vi "Host_timing_study.vi"() -> ()   [LabVIEW 2020]
uses:
  <vilib>/Analysis/7linalg.llb/Eigenvalue and Vectors Output Option.ctl
  <vilib>/Analysis/NI_AALPro.lvlib
  <vilib>/Analysis/7linalg.llb/Real Eigenvalues and Vectors.vi
  <vilib>/Analysis/NI_AALBase.lvlib
  <vilib>/Analysis/baseanly.llb/Real Inverse Matrix.vi
  <vilib>/rvi/interface/nirviMethod/nirviMethod.xnode
  <vilib>/Analysis/Matrix/NI_Matrix.lvlib
  <vilib>/Analysis/Matrix/Numeric/Multiply/Multiply - RM,RM.vi
  <vilib>/rvi/errors/niLvFpgaMergeErrorWithErrorCode.vi
  <vilib>/rvi/interface/nirviOpenFPGA/nirviOpenFPGA.xnode
  <vilib>/rvi/interface/nirviCloseFPGA/nirviCloseFPGA.xnode
  <vilib>/FPGAPlugInAG/Dynamic/niLvFpga_Close_Dynamic.vi
  <vilib>/Analysis/baseanly.llb/Matrix Type of Inverse Matrix.ctl
  FPGA Bitfiles/Cholesky_SGL_19_nodes.lvbitx
  <vilib>/FPGAPlugInAG/Dynamic/niLvFpga_Run_Dynamic.vi
  <vilib>/Analysis/Matrix/Numeric/Add/Add - RM,RM.vi
  <vilib>/addons/Multicore Analysis and Sparse Matrix/Linear Algebra/_linalg/Eigenvalues and Vectors_Output Option.ctl
  <vilib>/addons/Multicore Analysis and Sparse Matrix/Linear Algebra/_linalg/Eigenvalues and Vectors_Matrix Type (Real).ctl
  <vilib>/addons/Multicore Analysis and Sparse Matrix/Linear Algebra/_linalg/Eigenvalues and Vectors (DBL).vi
  <vilib>/addons/Multicore Analysis and Sparse Matrix/Linear Algebra/_linalg/Inverse Matrix (DBL).vi
  <vilib>/addons/Multicore Analysis and Sparse Matrix/Linear Algebra/_linalg/Inverse Matrix_Matrix Type.ctl
  <vilib>/addons/Multicore Analysis and Sparse Matrix/Linear Algebra/_linalg/Transpose Matrix (DBL).vi
  <vilib>/Analysis/Matrix/Numeric/Conversions/Array To Matrix - RA2.vi
  <vilib>/addons/Multicore Analysis and Sparse Matrix/Linear Algebra/_linalg/Cholesky Decomposition (DBL).vi
  <vilib>/Analysis/7linalg.llb/Real Cholesky Factorization.vi
  <vilib>/addons/Multicore Analysis and Sparse Matrix/Linear Algebra/_linalg/Generalized Eigenvalues and Vectors (DBL).vi
  <vilib>/Analysis/7linalg.llb/Real Generalized Eigenvalues and Vectors.vi
  FPGA Bitfiles/cholesky_SGL_CCL_19_nodes_v3.lvbitx
  <vilib>/FPGAPlugInAG/Dynamic/niLvFpga_WriteFifo_Dynamic.vi
  <vilib>/FPGAPlugInAG/Dynamic/niLvFpga_ReadFifo_Dynamic.vi
panel:
  out "Data":sgl[](array[numeric])
  out "Real 2D Array":dbl[][](array[numeric])
  in  "Enum":T1(ring)
  out "Eigenvalues":cdb[](array[numeric])
  out "eigenvalue solver (ms)":dbl
  out "preprocessing (ms)":dbl
  out "total run time (ms)":dbl
  out "Frequencies":dbl[](array[numeric])
  out "K input":dbl[][](array[numeric])
  out "M input":dbl[][](array[numeric])
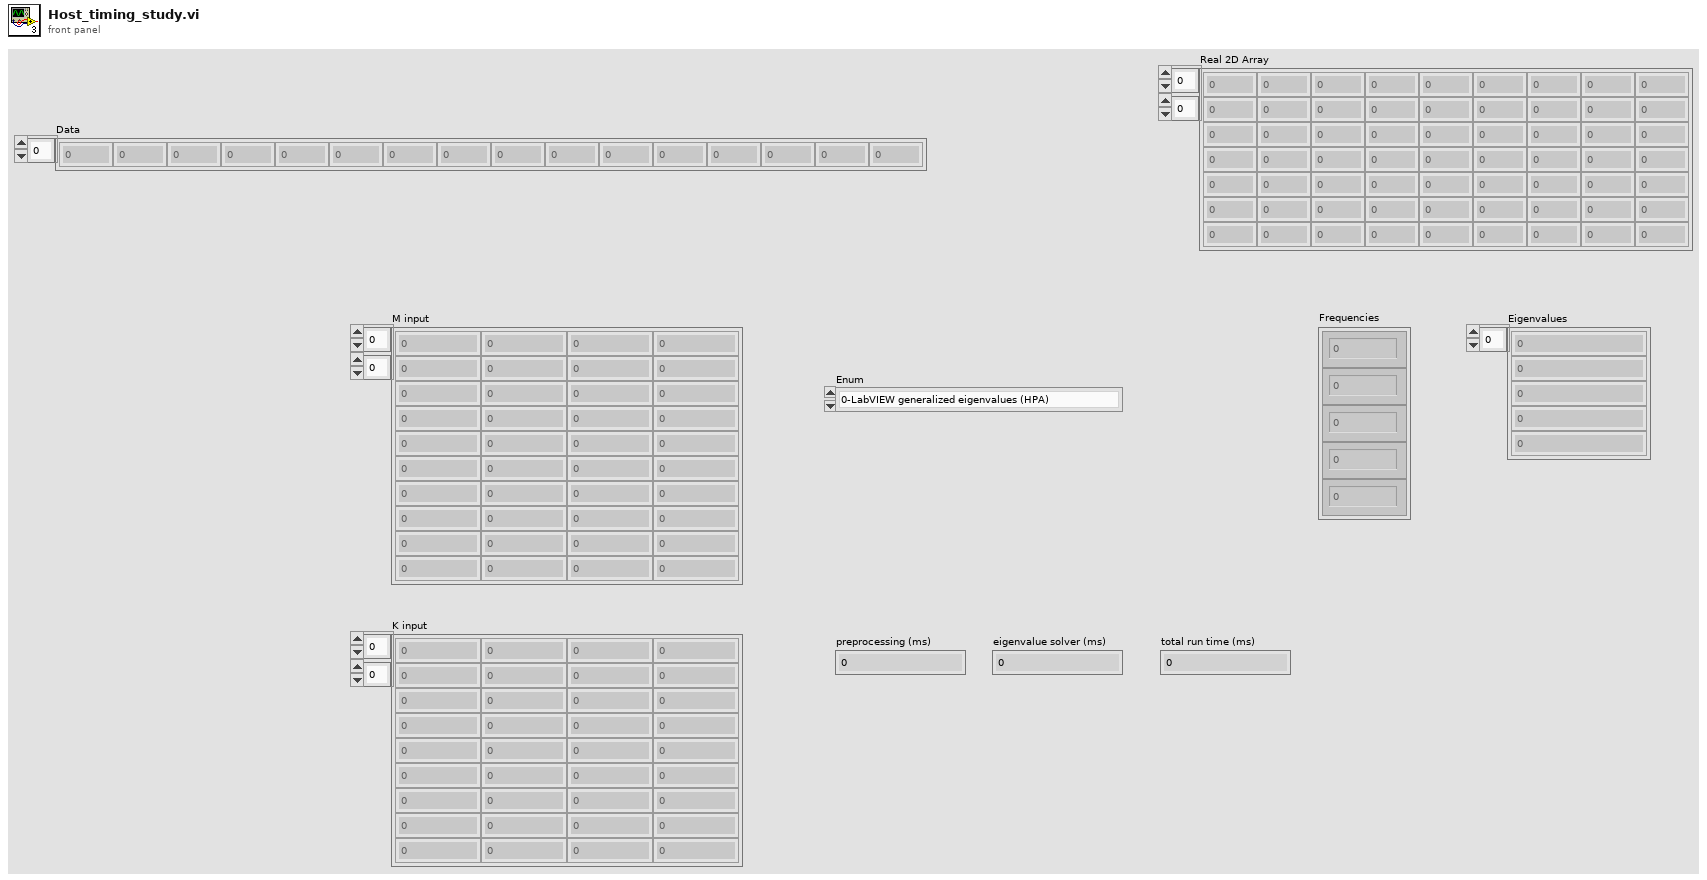
[diagram p1: front panel]
types:
  T1 = enum16{"0-LabVIEW generalized eigenvalues (HPA)", "1-LabVIEW generalized eigenvalues", "2-LabVIEW M^-1K eigenvalues (HPA)", "3-LabVIEW M^-1K eigenvalues", "4-LabVIEW Cholesky Factorization (HPA)", "5-LabVIEW Cholesky Factorization", "6-Cholesky Factorization CPU SGL", "7-Cholesky Factorization CPU FXP", "8-Cholesky Factorization FPGA SGL", "9-Cholesky Factorization FPGA SGL SCL"}
  T2 = typedef "NI_AALBase.lvlib/Matrix Type of Inverse Matrix.ctl" = enum32{"General", "Positive Definite", "Lower Triangular", "Upper Triangular"}
  T3 = typedef "NI_MASM_MtrxDecomposition.lvlib/Eigenvalues and Vectors_Output Option.ctl" = i32
  T4 = typedef "NI_Matrix.lvlib/RealMatrix.ctl" = dbl[][]
  T5 = typedef "NI_AALPro.lvlib/Eigenvalue and Vectors Output Option.ctl" = i32
  T6 = typedef "NI_MASM_BasicLinAlg.lvlib/Inverse Matrix_Matrix Type.ctl" = i32
  T7 = typedef "NI_MASM_MtrxDecomposition.lvlib/Eigenvalues and Vectors_Matrix Type (Real).ctl" = i32
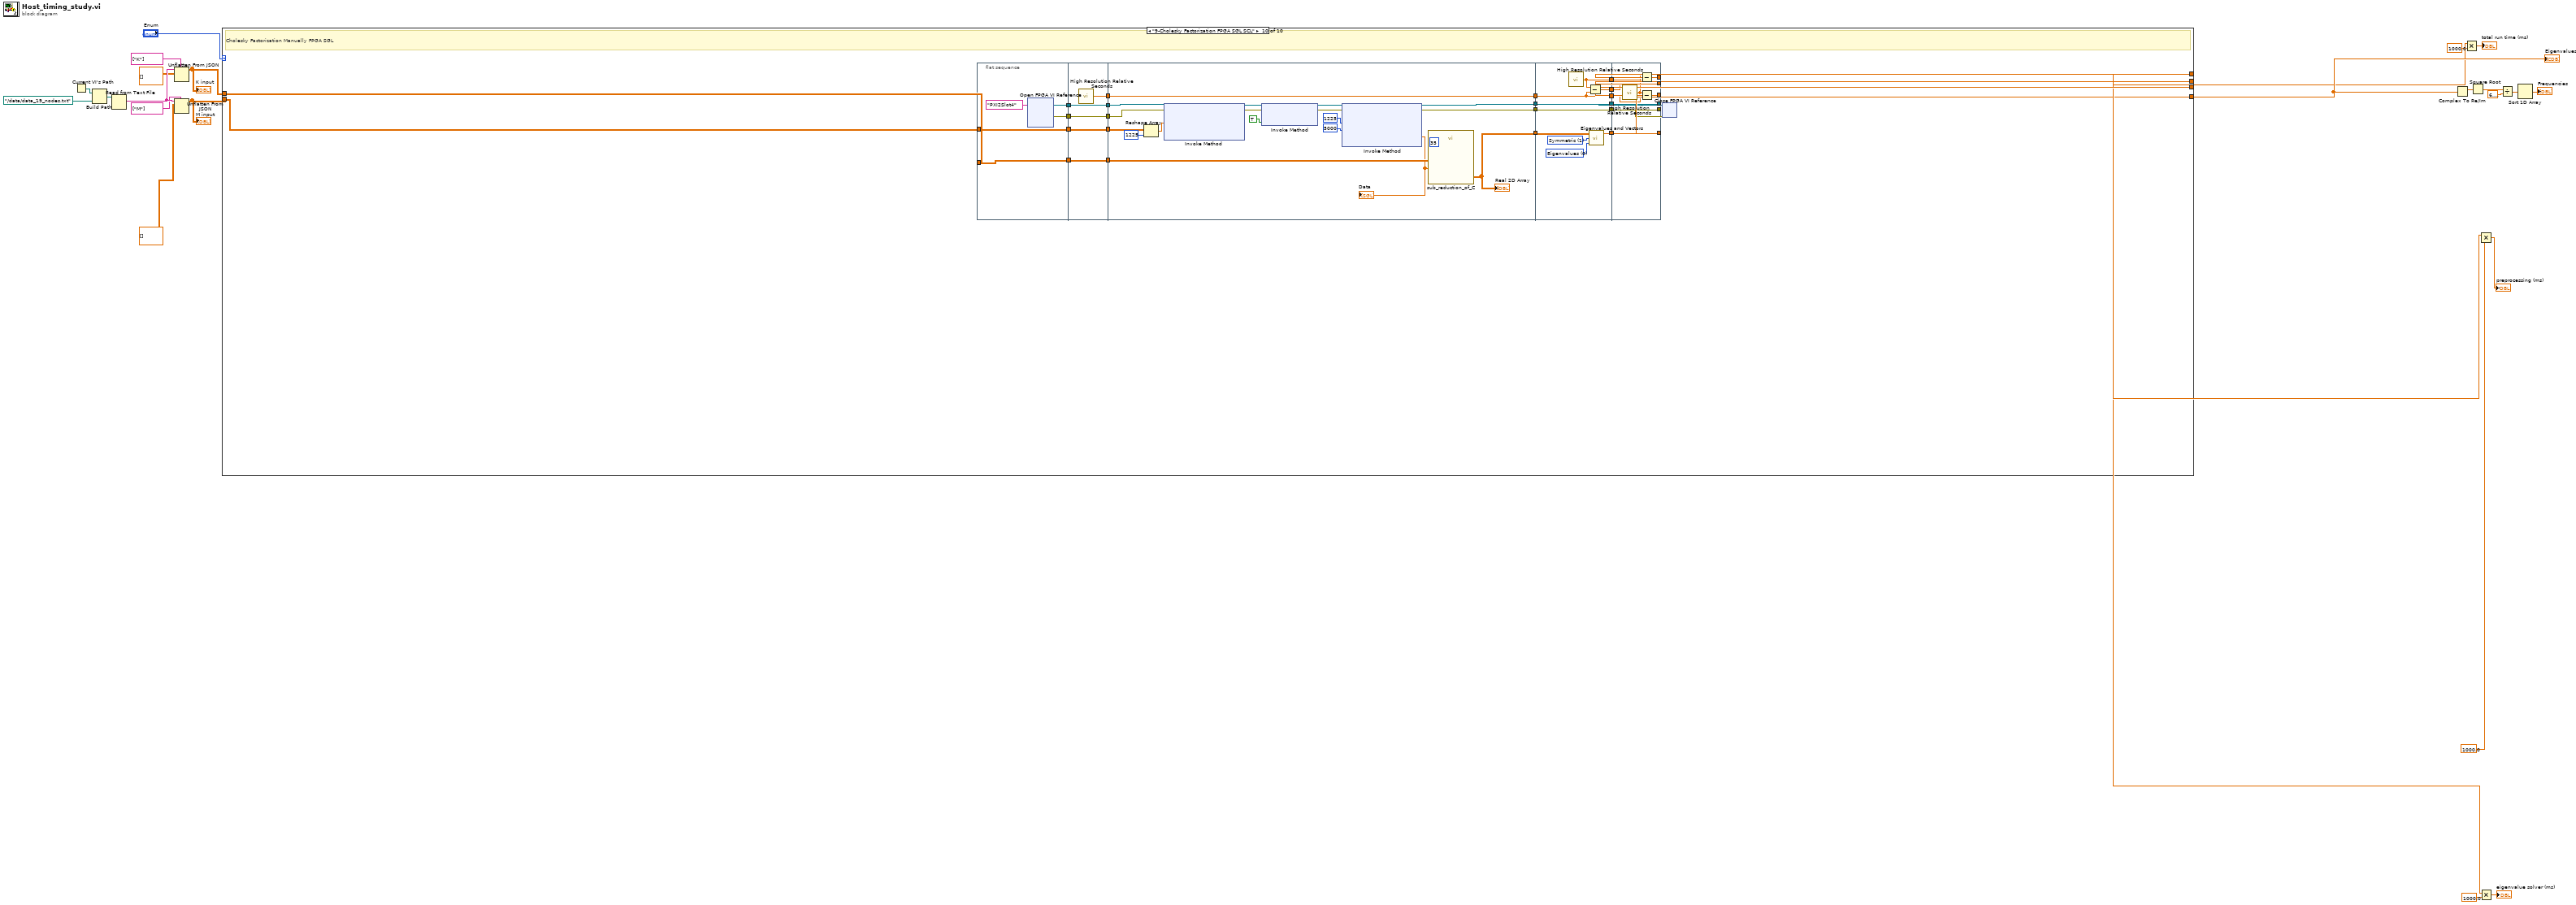
[diagram p0: block diagram]
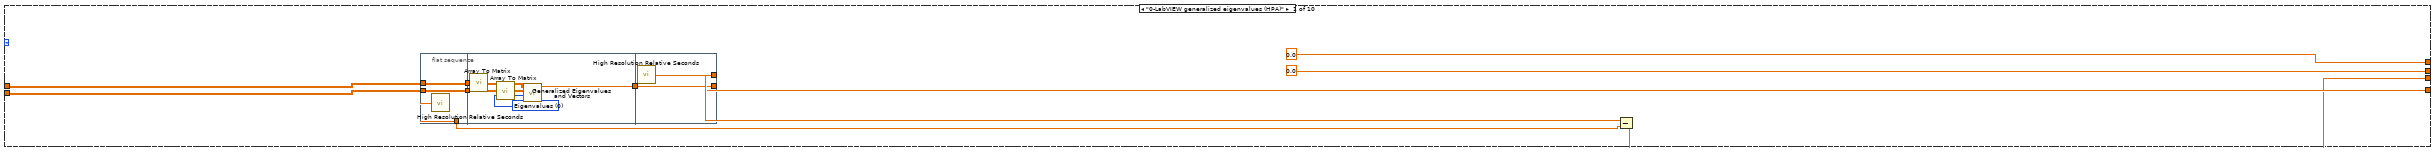
[diagram p2: hidden frame]
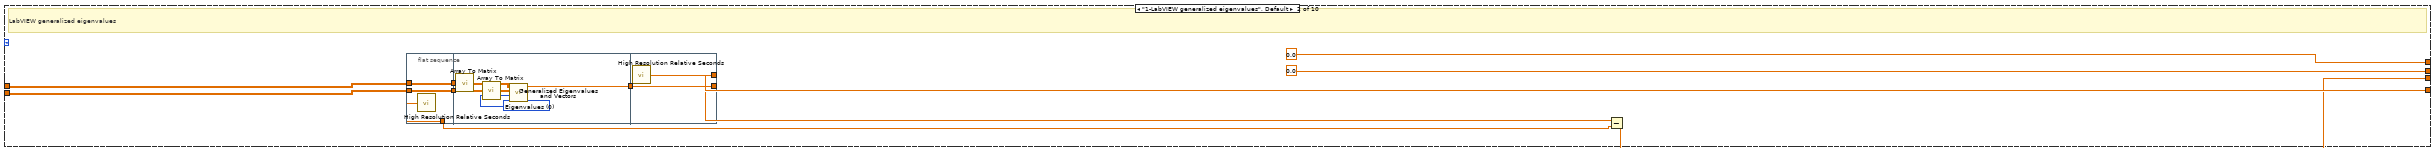
[diagram p3: hidden frame]
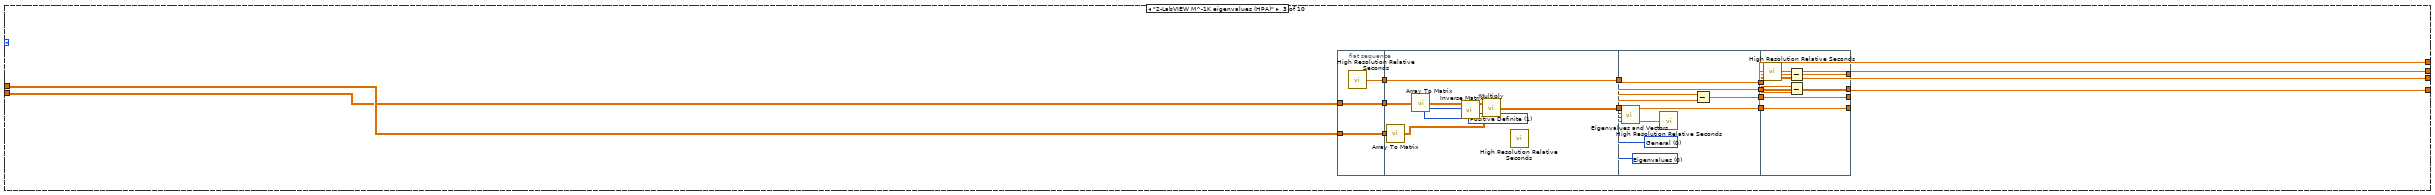
[diagram p4: hidden frame]
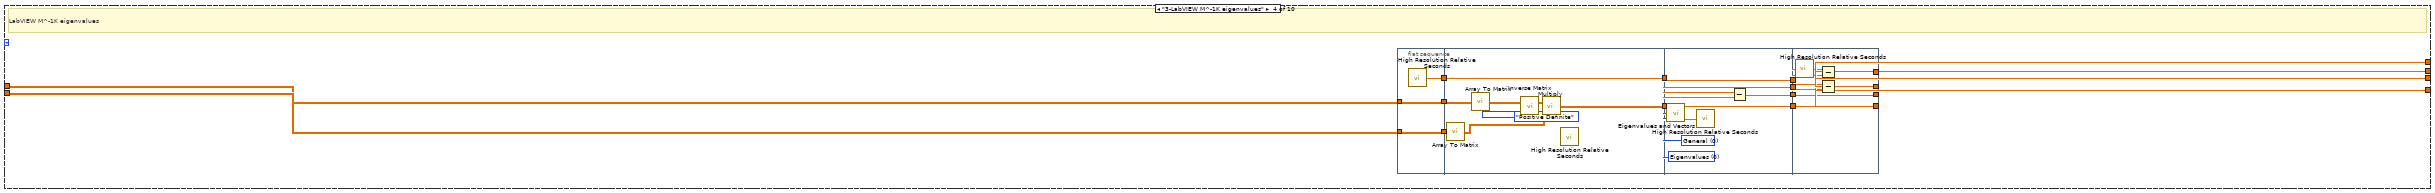
[diagram p5: hidden frame]
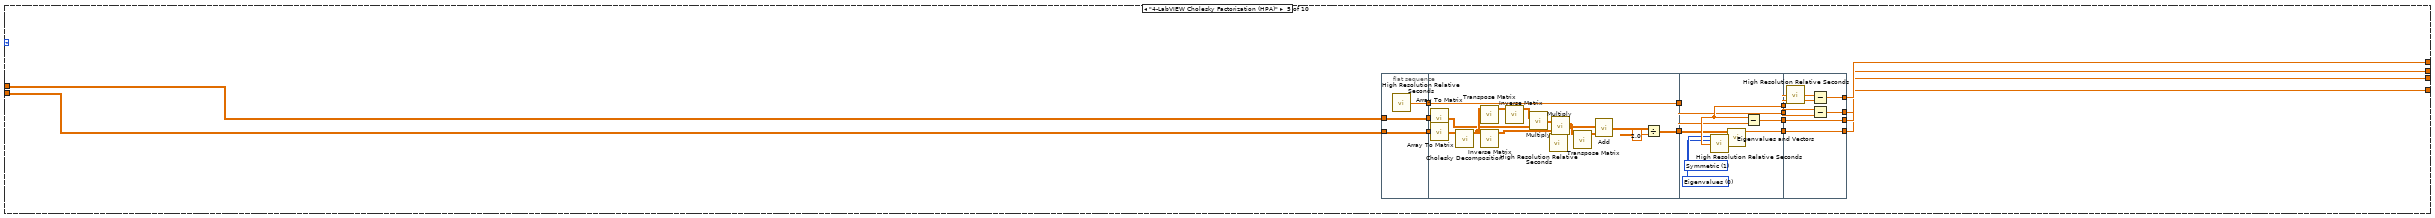
[diagram p6: hidden frame]
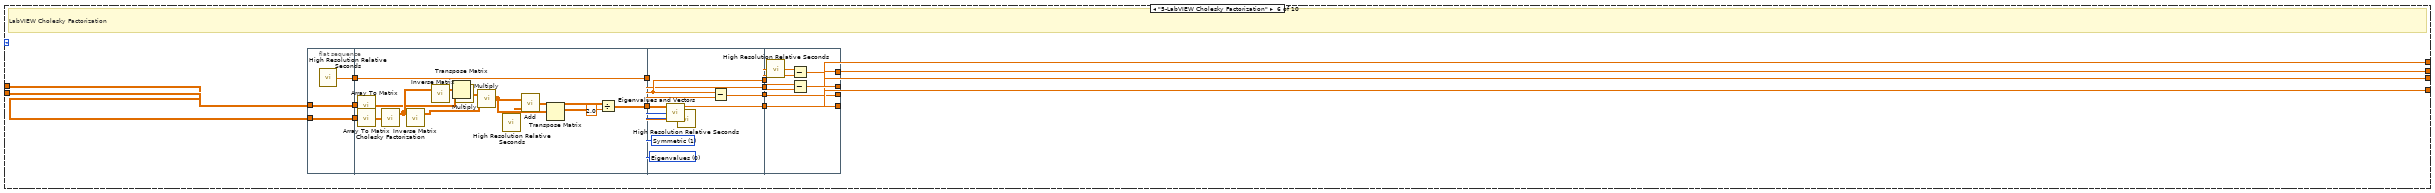
[diagram p7: hidden frame]
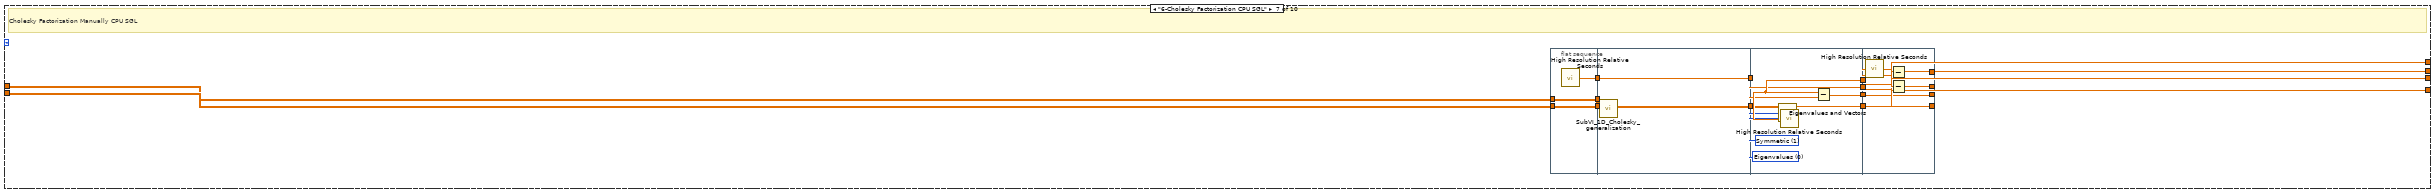
[diagram p8: hidden frame]
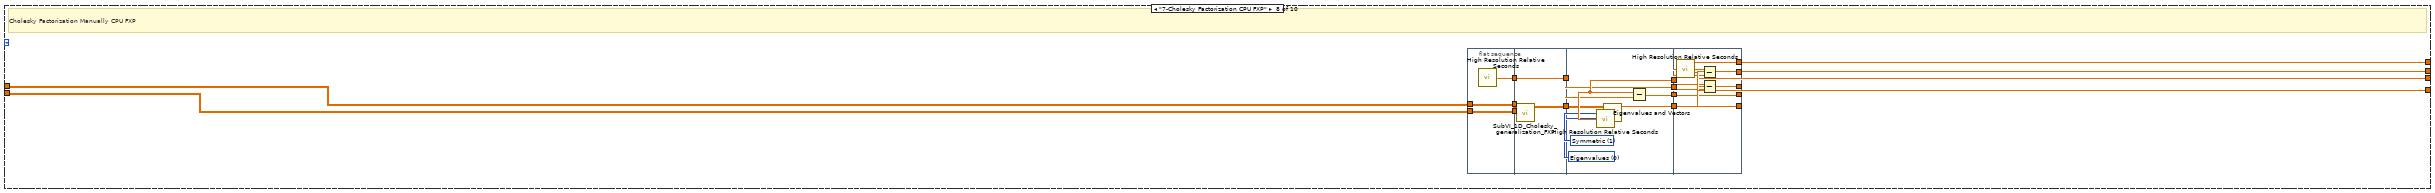
[diagram p9: hidden frame]
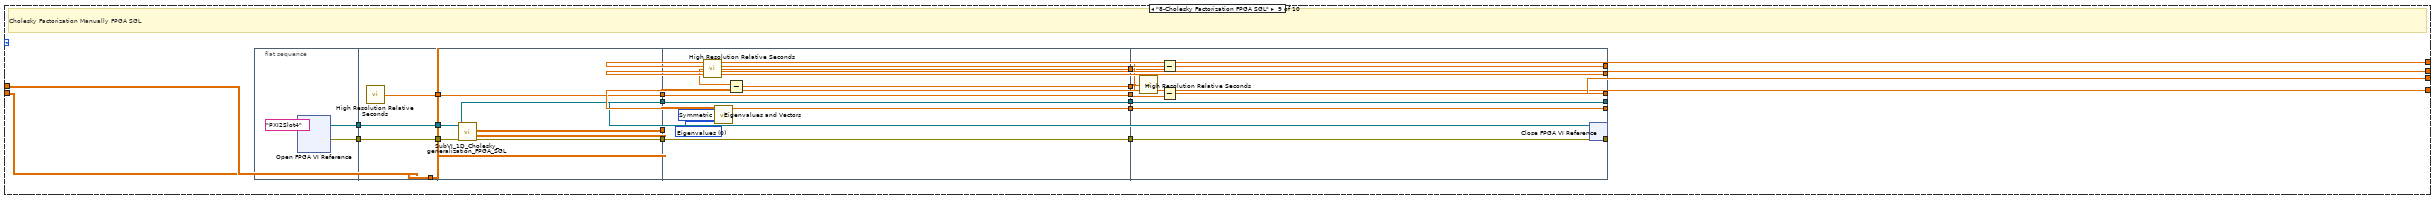
[diagram p10: hidden frame]
diagram:
  n1 = Current VI's Path() -> (path=w17:path)
  n2 = Build Path(base path=w17, name or relative path=path "../data/data_19_nodes.txt") -> (appended path=w16:path)
  n3 = Read from Text File(file (use dialog)=w16) -> (text=w23:string)  [unwired: 3 in, 3 out]
  n4 = Unflatten From JSON(path=string[] ["K"], JSON string=w23, type and defaults=dbl[][] []) -> (value=w25:dbl[][])  [unwired: 4 in, 1 out]
  "K input" <- w25
  n5 = Unflatten From JSON(path=string[] ["M"], JSON string=w23, type and defaults=dbl[][] []) -> (value=w26:dbl[][])  [unwired: 4 in, 1 out]
  "M input" <- w26
  n6 = case shown="\"9-Cholesky Factorization FPGA SGL SCL\"" "Enum" {
    tunnel: [w30 w59 w76 w125 w151 w207 w248 w284 w327 w388] -> w24
    tunnel: w26 -> [w31 w58 w71 w120 w155 w212 w254 w285 w332 w383]
    tunnel: w25 -> [w32 w57 w72 w117 w156 w211 w251 w286 w333 w376]
    tunnel: [w28 w51 w73 w121 w152 w204 w247 w281 w328 w389] -> w10
    tunnel: [0.0 0.0 w75 w114 w153 w201 w246 w282 w329 w390] -> w3
    tunnel: [0.0 0.0 w74 w111 w154 w198 w245 w283 w330 w391] -> w2
    frame "0-LabVIEW generalized eigenvalues (HPA)" {
      n7 = flat-sequence {
        tunnel: w32 -> [w39]
        tunnel: w31 -> [w40]
        tunnel: [w40] -> w37
        tunnel: [w39] -> w36
        tunnel: [w38] -> w33
        tunnel: w37 -> [w42]
        tunnel: w36 -> [w44]
        tunnel: [w45] -> w35
        tunnel: [w48] -> w30
        tunnel: w35 -> [w48]
        tunnel: [w47] -> w34
        frame #0 {
          n8 = call <vilib>:"High Resolution Relative Seconds.vi"() -> ("relative seconds"=w38:dbl)
        }
        frame #1 {
          w46 = T3 0 items=["Eigenvalues", "Eigenvalues & Vectors"] ("output option")
          n9 = call-poly <vilib>:"Array To Matrix.vi"("Real 2D Array"=w44) -> ("Real Matrix"=w43:T4)
          n10 = call-poly <vilib>:"Array To Matrix.vi"("Real 2D Array"=w42) -> ("Real Matrix"=w41:T4)
          n11 = call-poly <vilib>:"Generalized Eigenvalues and Vectors.vi"("output option"=w46, "B"=w41, "A"=w43) -> ("Eigenvalues"=w45:cdb[])  [unwired: 6 in, 2 out]
        }
        frame #2 {
          n12 = call <vilib>:"High Resolution Relative Seconds.vi"() -> ("relative seconds"=w47:dbl)
        }
      }
      n13 = Subtract(x=w34, y=w33) -> (x-y=w28:dbl)
    }
    frame "1-LabVIEW generalized eigenvalues", Default {
      # "LabVIEW generalized eigenvalues"
      n14 = flat-sequence {
        tunnel: w57 -> [w61]
        tunnel: w58 -> [w62]
        tunnel: [w62] -> w56
        tunnel: [w61] -> w55
        tunnel: [w60] -> w52
        tunnel: w56 -> [w65]
        tunnel: w55 -> [w66]
        tunnel: [w67] -> w54
        tunnel: [w70] -> w59
        tunnel: w54 -> [w70]
        tunnel: [w69] -> w53
        frame #0 {
          n15 = call <vilib>:"High Resolution Relative Seconds.vi"() -> ("relative seconds"=w60:dbl)
        }
        frame #1 {
          w68 = T5 0 items=["Eigenvalues", "Eigenvalues & Vectors"] ("output option")
          n16 = call-poly <vilib>:"Array To Matrix.vi"("Real 2D Array"=w66) -> ("Real Matrix"=w64:T4)
          n17 = call-poly <vilib>:"Array To Matrix.vi"("Real 2D Array"=w65) -> ("Real Matrix"=w63:T4)
          n18 = call-poly <vilib>:"Generalized Eigenvalues and Vectors.vi"("output option"=w68, "B"=w63, "A"=w64) -> ("Eigenvalues"=w67:cdb[])  [unwired: 3 in, 2 out]
        }
        frame #2 {
          n19 = call <vilib>:"High Resolution Relative Seconds.vi"() -> ("relative seconds"=w69:dbl)
        }
      }
      n20 = Subtract(x=w53, y=w52) -> (x-y=w51:dbl)
    }
    frame "2-LabVIEW M^-1K eigenvalues (HPA)" {
      n21 = flat-sequence {
        tunnel: w71 -> [w88]
        tunnel: [w88] -> w85
        tunnel: w72 -> [w87]
        tunnel: [w87] -> w84
        tunnel: [w86] -> w83
        tunnel: [w96] -> w82
        tunnel: w85 -> [w90]
        tunnel: w84 -> [w92]
        tunnel: w83 -> [w95]
        tunnel: [w95] -> w81
        tunnel: w82 -> [w103]
        tunnel: [w102] -> w80
        tunnel: [w99] -> w79
        tunnel: w81 -> [w99]
        tunnel: [w101] -> w78
        tunnel: [w100] -> w77
        tunnel: [w110] -> w76
        tunnel: w80 -> [w110]
        tunnel: w79 -> [w109]
        tunnel: [w108] -> w73
        tunnel: [w107] -> w75
        tunnel: w78 -> [w107]
        tunnel: w77 -> [w105]
        tunnel: [w104] -> w74
        frame #0 {
          n22 = call <vilib>:"High Resolution Relative Seconds.vi"() -> ("relative seconds"=w86:dbl)
        }
        frame #1 {
          w93 = T6 1 items=["General", "Positive Definite", "Lower Triangular", "Upper Triangular"] ("matrix type")
          n23 = call-poly <vilib>:"Array To Matrix.vi"("Real 2D Array"=w92) -> ("Real Matrix"=w91:T4)
          n24 = call-poly <vilib>:"Array To Matrix.vi"("Real 2D Array"=w90) -> ("Real Matrix"=w89:T4)
          n25 = call-poly <vilib>:"Inverse Matrix.vi"("matrix type"=w93, "Input Matrix"=w89) -> ("Inverse Matrix"=w94:T4)  [unwired: 8 in, 1 out]
          n26 = call-poly <vilib>:"Multiply.vi"("Real Matrix B"=w91, "Real Matrix A"=w94) -> ("A * B"=w96:T4)
          n27 = call <vilib>:"High Resolution Relative Seconds.vi"() -> ()  [unwired: 1 out]
        }
        frame #2 {
          w97 = T3 0 items=["Eigenvalues", "Eigenvalues & Vectors"] ("output option")
          w98 = T7 0 items=["General", "Symmetric"] ("matrix type")
          n28 = call-poly <vilib>:"Eigenvalues and Vectors.vi"("output option"=w97, "matrix type"=w98, "Input Matrix"=w103) -> ("Eigenvalues"=w102:cdb[])  [unwired: 6 in, 2 out]
          n29 = call <vilib>:"High Resolution Relative Seconds.vi"() -> ("relative seconds"=w100:dbl)
          n30 = Subtract(x=w100, y=w99) -> (x-y=w101:dbl)
        }
        frame #3 {
          n31 = call <vilib>:"High Resolution Relative Seconds.vi"() -> ("relative seconds"=w106:dbl)
          n32 = Subtract(x=w106, y=w105) -> (x-y=w104:dbl)
          n33 = Subtract(x=w106, y=w109) -> (x-y=w108:dbl)
        }
      }
    }
    frame "3-LabVIEW M^-1K eigenvalues" {
      # "LabVIEW M^-1K eigenvalues"
      n34 = flat-sequence {
        tunnel: w120 -> [w128]
        tunnel: [w128] -> w119
        tunnel: w117 -> [w127]
        tunnel: [w127] -> w118
        tunnel: [w126] -> w116
        tunnel: [w134] -> w124
        tunnel: w119 -> [w130]
        tunnel: w118 -> [w132]
        tunnel: w116 -> [w133]
        tunnel: [w133] -> w115
        tunnel: w124 -> [w143]
        tunnel: [w140] -> w123
        tunnel: [w137] -> w122
        tunnel: w115 -> [w137]
        tunnel: [w139] -> w113
        tunnel: [w138] -> w112
        tunnel: [w150] -> w125
        tunnel: w123 -> [w150]
        tunnel: w122 -> [w149]
        tunnel: [w148] -> w121
        tunnel: [w147] -> w114
        tunnel: w113 -> [w147]
        tunnel: w112 -> [w145]
        tunnel: [w144] -> w111
        frame #0 {
          n35 = call <vilib>:"High Resolution Relative Seconds.vi"() -> ("relative seconds"=w126:dbl)
        }
        frame #1 {
          n36 = call-poly <vilib>:"Array To Matrix.vi"("Real 2D Array"=w132) -> ("Real Matrix"=w131:T4)
          n37 = call-poly <vilib>:"Array To Matrix.vi"("Real 2D Array"=w130) -> ("Real Matrix"=w129:T4)
          n38 = call-poly <vilib>:"Inverse Matrix.vi"("matrix type"=Matrix_Type_of_Inverse_Matrix."Positive Definite", "Input Matrix"=w129) -> ("Inverse Matrix"=w136:T4)  [unwired: 1 out]
          n39 = call-poly <vilib>:"Multiply.vi"("Real Matrix B"=w131, "Real Matrix A"=w136) -> ("A * B"=w134:T4)
          n40 = call <vilib>:"High Resolution Relative Seconds.vi"() -> ()  [unwired: 1 out]
        }
        frame #2 {
          w141 = T5 0 items=["Eigenvalues", "Eigenvalues & Vectors"] ("output option")
          w142 = 0 items=["General", "Symmetric"] ("matrix type")
          n41 = call-poly <vilib>:"Eigenvalues and Vectors.vi"("output option"=w141, "matrix type"=w142, "Input Matrix"=w143) -> ("Eigenvalues"=w140:cdb[])  [unwired: 2 out]
          n42 = call <vilib>:"High Resolution Relative Seconds.vi"() -> ("relative seconds"=w138:dbl)
          n43 = Subtract(x=w138, y=w137) -> (x-y=w139:dbl)
        }
        frame #3 {
          n44 = call <vilib>:"High Resolution Relative Seconds.vi"() -> ("relative seconds"=w146:dbl)
          n45 = Subtract(x=w146, y=w145) -> (x-y=w144:dbl)
          n46 = Subtract(x=w146, y=w149) -> (x-y=w148:dbl)
        }
      }
    }
    frame "4-LabVIEW Cholesky Factorization (HPA)" {
      n47 = flat-sequence {
        tunnel: w156 -> [w167]
        tunnel: w155 -> [w168]
        tunnel: [w168] -> w165
        tunnel: [w167] -> w164
        tunnel: [w166] -> w163
        tunnel: w165 -> [w172]
        tunnel: w164 -> [w170]
        tunnel: [w180] -> w162
        tunnel: w163 -> [w179]
        tunnel: [w179] -> w161
        tunnel: w162 -> [w187]
        tunnel: [w186] -> w160
        tunnel: [w188] -> w159
        tunnel: w161 -> [w188]
        tunnel: [w190] -> w158
        tunnel: [w189] -> w157
        tunnel: [w197] -> w151
        tunnel: w160 -> [w197]
        tunnel: w159 -> [w196]
        tunnel: [w195] -> w152
        tunnel: [w194] -> w153
        tunnel: w158 -> [w194]
        tunnel: w157 -> [w192]
        tunnel: [w191] -> w154
        frame #0 {
          n48 = call <vilib>:"High Resolution Relative Seconds.vi"() -> ("relative seconds"=w166:dbl)
        }
        frame #1 {
          n49 = call-poly <vilib>:"Array To Matrix.vi"("Real 2D Array"=w170) -> ("Real Matrix"=w169:T4)
          n50 = call-poly <vilib>:"Array To Matrix.vi"("Real 2D Array"=w172) -> ("Real Matrix"=w171:T4)
          n51 = call-poly <vilib>:"Cholesky Decomposition.vi"("A"=w171) -> ("Cholesky"=w176:T4)  [unwired: 9 in, 1 out]
          n52 = call-poly <vilib>:"Transpose Matrix.vi"("Input Matrix"=w176) -> ("Matrix Transpose"=w175:T4)  [unwired: 9 in, 1 out]
          n53 = call-poly <vilib>:"Inverse Matrix.vi"("Input Matrix"=w176) -> ("Inverse Matrix"=w182:T4)  [unwired: 9 in, 1 out]
          n54 = call-poly <vilib>:"Inverse Matrix.vi"("Input Matrix"=w175) -> ("Inverse Matrix"=w183:T4)  [unwired: 9 in, 1 out]
          n55 = call-poly <vilib>:"Multiply.vi"("Real Matrix B"=w169, "Real Matrix A"=w183) -> ("A * B"=w181:T4)
          n56 = call <vilib>:"High Resolution Relative Seconds.vi"() -> ()  [unwired: 1 out]
          n57 = call-poly <vilib>:"Multiply.vi"("Real Matrix B"=w182, "Real Matrix A"=w181) -> ("A * B"=w174:T4)
          n58 = call-poly <vilib>:"Transpose Matrix.vi"("Input Matrix"=w174) -> ("Matrix Transpose"=w173:T4)  [unwired: 9 in, 1 out]
          n59 = call-poly <vilib>:"Add.vi"("Real Matrix B"=w173, "Real Matrix A"=w174) -> ("A + B"=w177:T4)
          n60 = Divide(x=w177, y=2.0) -> (x/y=w180:T4)
        }
        frame #2 {
          w184 = T3 0 items=["Eigenvalues", "Eigenvalues & Vectors"] ("output option")
          w185 = T7 1 items=["General", "Symmetric"] ("matrix type")
          n61 = call <vilib>:"High Resolution Relative Seconds.vi"() -> ("relative seconds"=w189:dbl)
          n62 = call-poly <vilib>:"Eigenvalues and Vectors.vi"("output option"=w184, "matrix type"=w185, "Input Matrix"=w187) -> ("Eigenvalues"=w186:cdb[])  [unwired: 6 in, 2 out]
          n63 = Subtract(x=w189, y=w188) -> (x-y=w190:dbl)
        }
        frame #3 {
          n64 = call <vilib>:"High Resolution Relative Seconds.vi"() -> ("relative seconds"=w193:dbl)
          n65 = Subtract(x=w193, y=w192) -> (x-y=w191:dbl)
          n66 = Subtract(x=w193, y=w196) -> (x-y=w195:dbl)
        }
      }
    }
    frame "5-LabVIEW Cholesky Factorization" {
      # "LabVIEW Cholesky Factorization"
      n67 = flat-sequence {
        tunnel: w211 -> [w214]
        tunnel: w212 -> [w215]
        tunnel: [w215] -> w210
        tunnel: [w214] -> w209
        tunnel: [w213] -> w203
        tunnel: w210 -> [w219]
        tunnel: w209 -> [w217]
        tunnel: [w224] -> w208
        tunnel: w203 -> [w223]
        tunnel: [w223] -> w202
        tunnel: w208 -> [w237]
        tunnel: [w236] -> w206
        tunnel: [w233] -> w205
        tunnel: w202 -> [w233]
        tunnel: [w235] -> w200
        tunnel: [w234] -> w199
        tunnel: [w244] -> w207
        tunnel: w206 -> [w244]
        tunnel: w205 -> [w243]
        tunnel: [w242] -> w204
        tunnel: [w241] -> w201
        tunnel: w200 -> [w241]
        tunnel: w199 -> [w239]
        tunnel: [w238] -> w198
        frame #0 {
          n68 = call <vilib>:"High Resolution Relative Seconds.vi"() -> ("relative seconds"=w213:dbl)
        }
        frame #1 {
          n69 = call-poly <vilib>:"Array To Matrix.vi"("Real 2D Array"=w217) -> ("Real Matrix"=w216:T4)
          n70 = call-poly <vilib>:"Array To Matrix.vi"("Real 2D Array"=w219) -> ("Real Matrix"=w218:T4)
          n71 = call-poly <vilib>:"Cholesky Factorization.vi"("A"=w218) -> ("Cholesky"=w229:T4)  [unwired: 1 out]
          n72 = call-poly <vilib>:"Inverse Matrix.vi"("Input Matrix"=w229) -> ("Inverse Matrix"=w227:T4)  [unwired: 1 in, 1 out]
          n73 = Transpose Matrix(1:w229) -> (0:w230:T4)
          n74 = call-poly <vilib>:"Inverse Matrix.vi"("Input Matrix"=w230) -> ("Inverse Matrix"=w228:T4)  [unwired: 1 in, 1 out]
          n75 = call-poly <vilib>:"Multiply.vi"("Real Matrix B"=w216, "Real Matrix A"=w228) -> ("A * B"=w226:T4)
          n76 = call-poly <vilib>:"Multiply.vi"("Real Matrix B"=w227, "Real Matrix A"=w226) -> ("A * B"=w225:T4)
          n77 = call <vilib>:"High Resolution Relative Seconds.vi"() -> ()  [unwired: 1 out]
          n78 = Transpose Matrix(1:w225) -> (0:w222:T4)
          n79 = call-poly <vilib>:"Add.vi"("Real Matrix B"=w222, "Real Matrix A"=w225) -> ("A + B"=w220:T4)
          n80 = Divide(x=w220, y=2.0) -> (x/y=w224:T4)
        }
        frame #2 {
          w231 = T5 0 items=["Eigenvalues", "Eigenvalues & Vectors"] ("output option")
          w232 = 1 items=["General", "Symmetric"] ("matrix type")
          n81 = call-poly <vilib>:"Eigenvalues and Vectors.vi"("output option"=w231, "matrix type"=w232, "Input Matrix"=w237) -> ("Eigenvalues"=w236:cdb[])  [unwired: 2 out]
          n82 = call <vilib>:"High Resolution Relative Seconds.vi"() -> ("relative seconds"=w234:dbl)
          n83 = Subtract(x=w234, y=w233) -> (x-y=w235:dbl)
        }
        frame #3 {
          n84 = call <vilib>:"High Resolution Relative Seconds.vi"() -> ("relative seconds"=w240:dbl)
          n85 = Subtract(x=w240, y=w239) -> (x-y=w238:dbl)
          n86 = Subtract(x=w240, y=w243) -> (x-y=w242:dbl)
        }
      }
    }
    frame "6-Cholesky Factorization CPU SGL" {
      # "Cholesky Factorization Manually CPU SGL"
      n87 = flat-sequence {
        tunnel: [w262] -> w259
        tunnel: w254 -> [w261]
        tunnel: [w261] -> w253
        tunnel: [w260] -> w252
        tunnel: w251 -> [w260]
        tunnel: w259 -> [w266]
        tunnel: [w266] -> w258
        tunnel: w253 -> [w265]
        tunnel: w252 -> [w264]
        tunnel: [w263] -> w250
        tunnel: [w269] -> w257
        tunnel: w258 -> [w269]
        tunnel: [w273] -> w256
        tunnel: [w272] -> w255
        tunnel: w250 -> [w271]
        tunnel: [w270] -> w249
        tunnel: [w274] -> w248
        tunnel: w257 -> [w280]
        tunnel: [w279] -> w247
        tunnel: [w278] -> w246
        tunnel: w256 -> [w278]
        tunnel: w255 -> [w276]
        tunnel: [w275] -> w245
        tunnel: w249 -> [w274]
        frame #0 {
          n88 = call <vilib>:"High Resolution Relative Seconds.vi"() -> ("relative seconds"=w262:dbl)
        }
        frame #1 {
          n89 = call "SubVI_1D_Cholesky_generalization.vi"("K"=w264, "M"=w265) -> ("C"=w263:dbl[][])  [unwired: 9 in]
        }
        frame #2 {
          w267 = T5 0 items=["Eigenvalues", "Eigenvalues & Vectors"] ("output option")
          w268 = 1 items=["General", "Symmetric"] ("matrix type")
          n90 = call-poly <vilib>:"Eigenvalues and Vectors.vi"("output option"=w267, "matrix type"=w268, "Input Matrix"=w271) -> ("Eigenvalues"=w270:cdb[])  [unwired: 2 out]
          n91 = call <vilib>:"High Resolution Relative Seconds.vi"() -> ("relative seconds"=w272:dbl)
          n92 = Subtract(x=w272, y=w269) -> (x-y=w273:dbl)
        }
        frame #3 {
          n93 = call <vilib>:"High Resolution Relative Seconds.vi"() -> ("relative seconds"=w277:dbl)
          n94 = Subtract(x=w277, y=w276) -> (x-y=w275:dbl)
          n95 = Subtract(x=w277, y=w280) -> (x-y=w279:dbl)
        }
      }
    }
    frame "7-Cholesky Factorization CPU FXP" {
      # "Cholesky Factorization Manually CPU FXP"
      n96 = flat-sequence {
        tunnel: [w298] -> w295
        tunnel: w286 -> [w297]
        tunnel: [w297] -> w294
        tunnel: [w296] -> w293
        tunnel: w285 -> [w296]
        tunnel: w295 -> [w302]
        tunnel: [w302] -> w292
        tunnel: w294 -> [w301]
        tunnel: w293 -> [w300]
        tunnel: [w299] -> w291
        tunnel: [w305] -> w290
        tunnel: w292 -> [w305]
        tunnel: [w309] -> w289
        tunnel: [w308] -> w288
        tunnel: w291 -> [w307]
        tunnel: [w306] -> w287
        tunnel: [w311] -> w284
        tunnel: w290 -> [w316]
        tunnel: [w315] -> w281
        tunnel: [w314] -> w282
        tunnel: w289 -> [w314]
        tunnel: w288 -> [w312]
        tunnel: [w310] -> _
        tunnel: w287 -> [w311]
        tunnel: [w310] -> w283
        frame #0 {
          n97 = call <vilib>:"High Resolution Relative Seconds.vi"() -> ("relative seconds"=w298:dbl)
        }
        frame #1 {
          n98 = call "SubVI_1D_Cholesky_generalization_FXP.vi"("M"=w300, "K"=w301) -> ("C"=w299:dbl[][])  [unwired: 9 in]
        }
        frame #2 {
          w303 = T5 0 items=["Eigenvalues", "Eigenvalues & Vectors"] ("output option")
          w304 = 1 items=["General", "Symmetric"] ("matrix type")
          n99 = call <vilib>:"High Resolution Relative Seconds.vi"() -> ("relative seconds"=w308:dbl)
          n100 = call-poly <vilib>:"Eigenvalues and Vectors.vi"("output option"=w303, "matrix type"=w304, "Input Matrix"=w307) -> ("Eigenvalues"=w306:cdb[])  [unwired: 2 out]
          n101 = Subtract(x=w308, y=w305) -> (x-y=w309:dbl)
        }
        frame #3 {
          n102 = call <vilib>:"High Resolution Relative Seconds.vi"() -> ("relative seconds"=w313:dbl)
          n103 = Subtract(x=w313, y=w312) -> (x-y=w310:dbl)
          n104 = Subtract(x=w313, y=w316) -> (x-y=w315:dbl)
        }
      }
    }
    frame "8-Cholesky Factorization FPGA SGL" {
      # "Cholesky Factorization Manually FPGA SGL"
      n105 = flat-sequence {
        tunnel: [w341] -> w326
        tunnel: [w340] -> w320
        tunnel: [w345] -> w339
        tunnel: w326 -> [w344]
        tunnel: [w344] -> w325
        tunnel: w320 -> [w343]
        tunnel: [w343] -> w319
        tunnel: w339 -> [w353]
        tunnel: [w353] -> w338
        tunnel: w333 -> [w352]
        tunnel: w332 -> [w351]
        tunnel: [w350] -> w331
        tunnel: w325 -> [w349]
        tunnel: [w348] -> w324
        tunnel: [w347] -> w322
        tunnel: w319 -> [w346]
        tunnel: [w360] -> w337
        tunnel: [w358] -> w336
        tunnel: w338 -> [w358]
        tunnel: [w362] -> w335
        tunnel: [w361] -> w334
        tunnel: w331 -> [w359]
        tunnel: w324 -> [w355]
        tunnel: [w355] -> w323
        tunnel: w322 -> [w354]
        tunnel: [w354] -> w321
        tunnel: [w371] -> w327
        tunnel: w337 -> [w371]
        tunnel: w336 -> [w370]
        tunnel: [w369] -> w328
        tunnel: [w368] -> w329
        tunnel: w335 -> [w368]
        tunnel: w334 -> [w366]
        tunnel: [w365] -> w330
        tunnel: w323 -> [w364]
        tunnel: w321 -> [w363]
        tunnel: [w364] -> w318
        tunnel: [w363] -> w317
        frame #0 {
          n106 = xnode "Open FPGA VI Reference"("resource name"=tag "PXI2Slot4") -> ("FPGA VI Reference Out"=w341:refnum<k20>, "error out"=w340:errorcluster)  [unwired: 1 in]
        }
        frame #1 {
          n107 = call <vilib>:"High Resolution Relative Seconds.vi"() -> ("relative seconds"=w345:dbl)
        }
        frame #2 {
          n108 = call "SubVI_1D_Cholesky_generalization_FPGA_SGL.vi"("error in (no error)"=w346, "M"=w351, "K"=w352, "Refnum in"=w349) -> ("error out"=w347:errorcluster, "C"=w350:dbl[][], "Refnum out"=w348:refnum<k20>)  [unwired: 5 in]
        }
        frame #3 {
          w356 = T5 0 items=["Eigenvalues", "Eigenvalues & Vectors"] ("output option")
          w357 = 1 items=["General", "Symmetric"] ("matrix type")
          n109 = call <vilib>:"High Resolution Relative Seconds.vi"() -> ("relative seconds"=w361:dbl)
          n110 = call-poly <vilib>:"Eigenvalues and Vectors.vi"("output option"=w356, "matrix type"=w357, "Input Matrix"=w359) -> ("Eigenvalues"=w360:cdb[])  [unwired: 2 out]
          n111 = Subtract(x=w361, y=w358) -> (x-y=w362:dbl)
        }
        frame #4 {
          n112 = call <vilib>:"High Resolution Relative Seconds.vi"() -> ("relative seconds"=w367:dbl)
          n113 = Subtract(x=w367, y=w366) -> (x-y=w365:dbl)
          n114 = Subtract(x=w367, y=w370) -> (x-y=w369:dbl)
        }
      }
      n115 = xnode "Close FPGA VI Reference"("FPGA VI Reference In"=w318, "error in"=w317) -> ()  [unwired: 1 out]
    }
    frame "9-Cholesky Factorization FPGA SGL SCL" {
      # "Cholesky Factorization Manually FPGA SGL"
      n116 = flat-sequence {
        tunnel: [w402] -> w386
        tunnel: [w401] -> w384
        tunnel: w383 -> [w401]
        tunnel: w376 -> [w400]
        tunnel: [w400] -> w375
        tunnel: [w399] -> w372
        tunnel: [w408] -> w398
        tunnel: [w407] -> w387
        tunnel: w386 -> [w407]
        tunnel: [w406] -> w385
        tunnel: w384 -> [w406]
        tunnel: w375 -> [w405]
        tunnel: [w405] -> w374
        tunnel: [w404] -> w373
        tunnel: w372 -> [w404]
        tunnel: w398 -> [w427]
        tunnel: [w427] -> w397
        tunnel: [w426] -> w396
        tunnel: w387 -> [w425]
        tunnel: w385 -> [w424]
        tunnel: [w423] -> w382
        tunnel: [w422] -> w378
        tunnel: w374 -> [w421]
        tunnel: w373 -> [w420]
        tunnel: [w434] -> w395
        tunnel: [w432] -> w394
        tunnel: w397 -> [w432]
        tunnel: [w436] -> w393
        tunnel: [w435] -> w392
        tunnel: w396 -> [w433]
        tunnel: w382 -> [w431]
        tunnel: [w431] -> w381
        tunnel: w378 -> [w430]
        tunnel: [w430] -> w377
        tunnel: [w445] -> w388
        tunnel: w395 -> [w445]
        tunnel: w394 -> [w444]
        tunnel: [w443] -> w389
        tunnel: [w442] -> w390
        tunnel: w393 -> [w442]
        tunnel: w392 -> [w440]
        tunnel: [w439] -> w391
        tunnel: w381 -> [w438]
        tunnel: [w438] -> w380
        tunnel: [w437] -> w379
        tunnel: w377 -> [w437]
        frame #0 {
          n117 = xnode "Open FPGA VI Reference"("resource name"=tag "PXI2Slot4") -> ("FPGA VI Reference Out"=w402:refnum<k20>, "error out"=w399:errorcluster)  [unwired: 1 in]
        }
        frame #1 {
          n118 = call <vilib>:"High Resolution Relative Seconds.vi"() -> ("relative seconds"=w408:dbl)
        }
        frame #2 {
          n119 = Reshape Array(w424, 1225 ("dimension size")) -> (w419:dbl[])
          n120 = xnode "Invoke Method"("FPGA VI Reference In"=w425, "error in"=w420, "Data"=w419) -> ("FPGA VI Reference Out"=w418:refnum<k20>, "error out"=w417:errorcluster)  [unwired: 1 in, 1 out]
          n121 = xnode "Invoke Method"("FPGA VI Reference In"=w418, "error in"=w417, "Wait Until Done (F)"=TRUE) -> ("FPGA VI Reference Out"=w416:refnum<k20>, "error out"=w415:errorcluster)
          n122 = xnode "Invoke Method"("FPGA VI Reference In"=w416, "error in"=w415, "Number of Elements"=u32 1225, "Timeout (ms)"=5000) -> ("FPGA VI Reference Out"=w423:refnum<k20>, "error out"=w422:errorcluster, "Data"=w414:sgl[])  [unwired: 1 out]
          "Data" <- w414
          n123 = call "sub_reduction_of_C.vi"("dimension size"=35, "L"=w414, "K"=w421) -> ("Real 2D Array"=w426:dbl[][])  [unwired: 8 in]
          "Real 2D Array" <- w426
        }
        frame #3 {
          w428 = T5 0 items=["Eigenvalues", "Eigenvalues & Vectors"] ("output option")
          w429 = 1 items=["General", "Symmetric"] ("matrix type")
          n124 = call <vilib>:"High Resolution Relative Seconds.vi"() -> ("relative seconds"=w435:dbl)
          n125 = Subtract(x=w435, y=w432) -> (x-y=w436:dbl)
          n126 = call-poly <vilib>:"Eigenvalues and Vectors.vi"("output option"=w428, "matrix type"=w429, "Input Matrix"=w433) -> ("Eigenvalues"=w434:cdb[])  [unwired: 2 out]
        }
        frame #4 {
          n127 = call <vilib>:"High Resolution Relative Seconds.vi"() -> ("relative seconds"=w441:dbl)
          n128 = Subtract(x=w441, y=w440) -> (x-y=w439:dbl)
          n129 = Subtract(x=w441, y=w444) -> (x-y=w443:dbl)
        }
      }
      n130 = xnode "Close FPGA VI Reference"("FPGA VI Reference In"=w380, "error in"=w379) -> ()  [unwired: 1 out]
    }
  }
  "Eigenvalues" <- w24
  n131 = Complex To Re/Im ("Complex To Cartesian.vi")(x + iy=w24) -> (x=w13:dbl[])  [unwired: 1 out]
  n132 = Multiply(x=w10, y=1000.0) -> (x*y=→"total run time (ms)":dbl)
  n133 = Square Root ("Square Root.vi")(x=w13) -> (sqrt(x)=w14:dbl[])
  n134 = Multiply(x=w3, y=1000.0) -> (x*y=→"preprocessing (ms)":dbl)
  n135 = Multiply(x=w2, y=1000.0) -> (x*y=→"eigenvalue solver (ms)":dbl)
  n136 = Divide(x=w14, y=6.283185307179586) -> (x/y=w15:dbl[])
  n137 = Sort 1D Array(array=w15) -> (sorted array=→"Frequencies":dbl[])
